vi "checkFinishKeeperPlay.vi"(8 "error in (no error)":errorcluster, 10 "Game":refnum<class "Game.lvclass">, 11 "KeeperPlay in":refnum<class "KeeperPlay.lvclass">) -> (0 "error out":errorcluster, 2 "Boolean":bool, 3 "KeeperPlay out":refnum<class "KeeperPlay.lvclass">)   [LabVIEW 2023, in "KeeperPlay.lvclass"]
uses:
  KeeperPlay.lvclass
  Game_class/Game.lvclass
  Referee_class/command_interpreted.ctl
  Game_class/Game.lvclass/Game.ctl
  Referee_class/Referee.lvclass/Referee.ctl
  Game_class/Read Referee.vi
  Referee_class/Read command_interpreted.vi
  Referee_class/Referee.lvclass
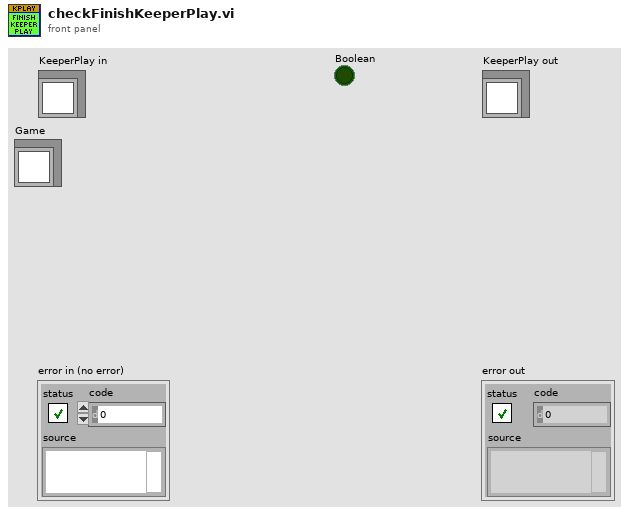
[diagram p1: front panel]
types:
  T1 = typedef "command_interpreted.ctl" = enum16{"Goal Ally", "Goal Enemy", "Ball Placement Enemy", "Ball Placement Ally", "Normal Half Time", "Extra Time  Break", "Extra Half Time", "None", "Post Game", "PKA Normal Start", "Prepare Kickoff Ally", "PKE Normal Start", "Prepare Kickoff Enemy", "Force Start", "Halt", "Timeout", "Prepare Penalty Ally", "Prepare Penalty Enemy", "PPA NormalStart", "PPE Normal Start", "Indirect Free Ally", "Direct Free Enemy", "Direct Free Ally", "Indirect Free Enemy", "Stop"}
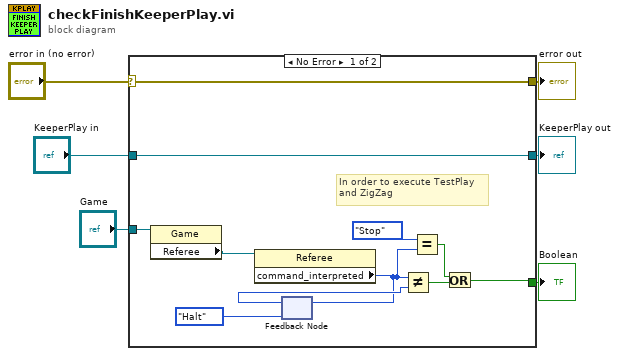
[diagram p0: block diagram]
diagram:
  n1 = case shown="No Error" "error in (no error)" {
    selector: "error in (no error)" -> [w16 w19]
    tunnel: [w16 w19] -> w5
    tunnel: [w17 w18] -> w3
    tunnel: "KeeperPlay in" -> [w17 w18]
    tunnel: "Game" -> [w15 _]
    tunnel: [w11 _] -> w1
    frame No Error {
      # "In order to execute TestPlay \nand ZigZag"
      n2 = property class="Game"(reference=w15) -> ("Referee"=w14:refnum<class "Referee.lvclass">)  [unwired: 1 in, 2 out]
      n3 = property class="Referee"(reference=w14) -> ("command_interpreted"=w8:T1)  [unwired: 1 in, 2 out]
      n4 = feedback-in #1(w8) -> ()
      n5 = feedback #1(command_interpreted."Halt" ("command_interpreted")) -> (w13:T1)
      n6 = Not Equal?(x=w8, y=w13) -> (x != y?=w10:bool)
      n7 = Equal?(x=command_interpreted."Stop", y=w8) -> (x = y?=w9:bool)
      n8 = Or(x=w9, y=w10) -> (x .or. y?=w11:bool)
    }
    frame Error {
    }
  }
  "error out" <- w5
  "KeeperPlay out" <- w3
  "Boolean" <- w1
